vi "IslandLines.vi"(6 "Spacing":dbl, 7 "IslandSize":dbl, 8 "yMax":dbl, 9 "yMin":dbl, 10 "xMax":dbl, 11 "xMin":dbl) -> (2 "Poly2D":T1, 3 "Pnts":sgl[][](array[numeric]))   [LabVIEW 2014]
uses:
  TypeDefs/Poly2DwSlope.ctl
  TypeDefs/Point2DwSlope.ctl
panel:
  out "XY Graph":T3(graph)
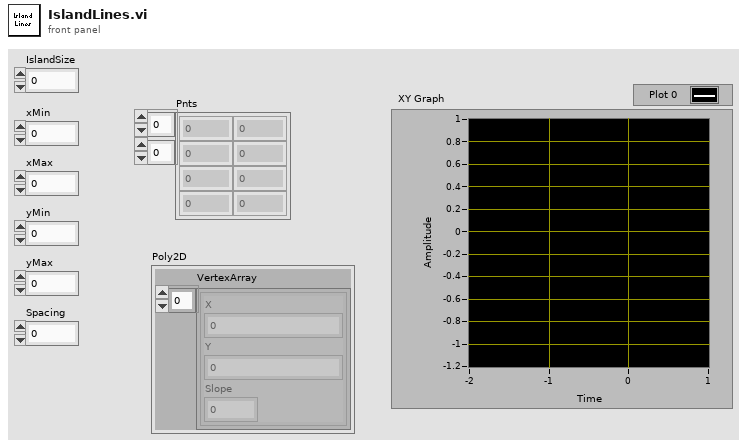
[diagram p1: front panel]
types:
  T1 = typedef "Poly2DwSlope.ctl" = cluster{"VertexArray":T2[]}
  T2 = typedef "Point2DwSlope.ctl" = cluster{"X":sgl, "Y":sgl, "Slope":dbl}
  T3 = cluster{"VertexArray":cluster{"X":sgl, "Y":sgl, "Slope":dbl}[]}[]
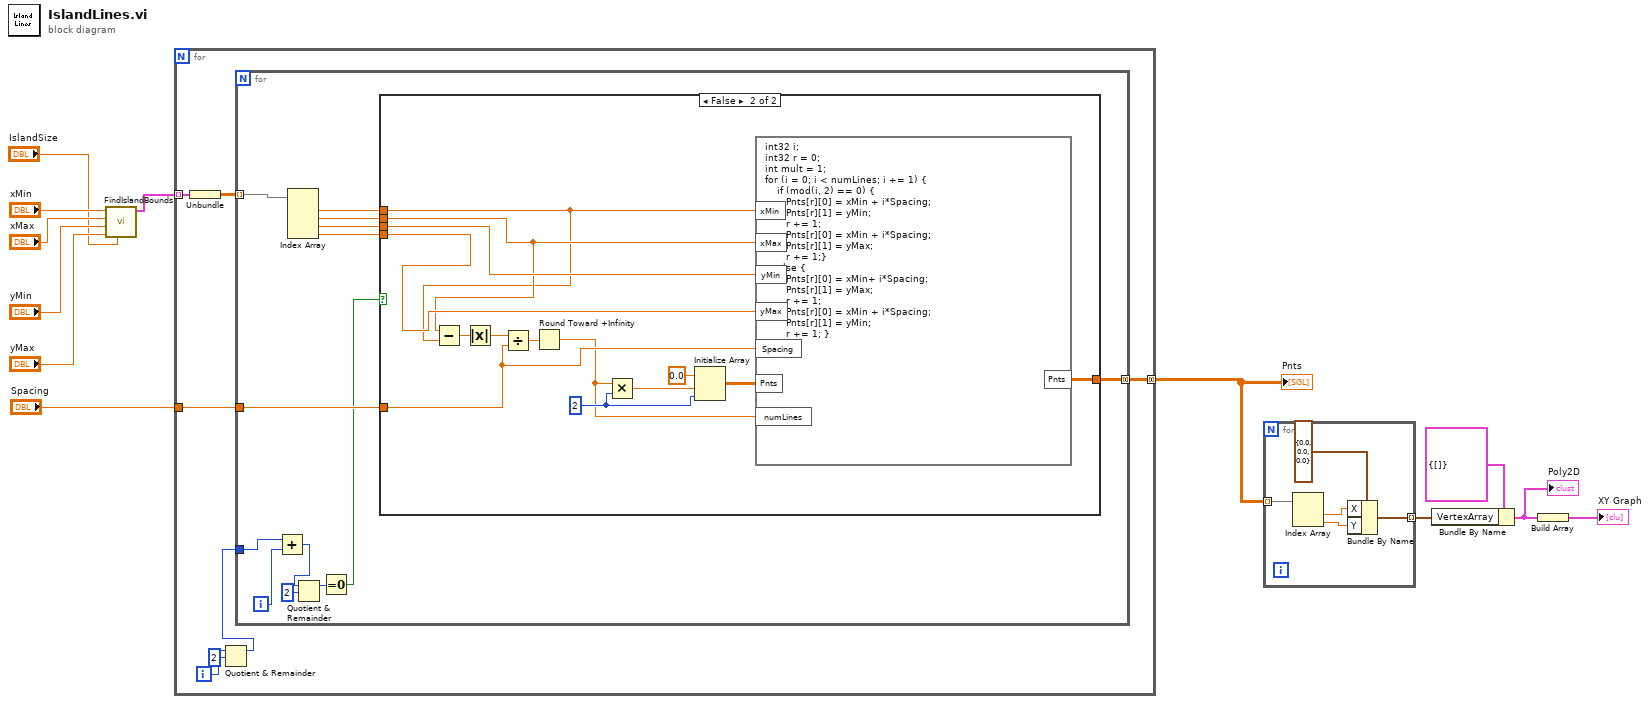
[diagram p0: block diagram]
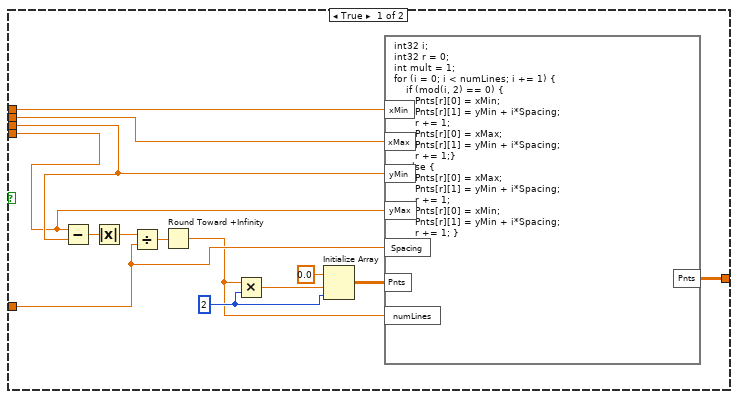
[diagram p2: hidden frame]
diagram:
  n1 = call "FindIslandBounds.vi"("IslandSize"="IslandSize", "yMax"="yMax", "yMin"="yMin", "xMax"="xMax", "xMin"="xMin") -> ("Bounds"=w2:cluster{dbl[][]}[])  [unwired: 6 in]
  n2 = for {
    tunnel: "Spacing" -> [w19]
    tunnel: [w18] -> w11 mode=concatenating
    tunnel: w2 -> [w17] mode=indexing
    i -> [w16]
    n3 = Unbundle(w17) -> (w14:dbl[][])
    n4 = Quotient & Remainder(x=w16, y=2) -> (x-y*floor(x/y)=w13:i32)  [unwired: 1 out]
    n5 = for {
      tunnel: w19 -> [w32]
      tunnel: [w31] -> w18 mode=concatenating
      tunnel: w14 -> [w30] mode=indexing
      tunnel: w13 -> [w21]
      i -> [w22]
      n6 = Add(x=w21, y=w22) -> (x+y=w20:i32)
      n7 = Index Array(array=w30) -> (element #1=w29:dbl, element #2=w28:dbl, element #3=w27:dbl, element #4=w26:dbl)  [unwired: 4 in]
      n8 = Quotient & Remainder(x=w20, y=2) -> (x-y*floor(x/y)=w25:i32)  [unwired: 1 out]
      n9 = Equal To 0?(x=w25) -> (x = 0?=w23:bool)
      n10 = case shown="False" w23 {
        tunnel: w32 -> [w39 w53]
        tunnel: [w37 w51] -> w31
        tunnel: w29 -> [w36 w47]
        tunnel: w28 -> [w35 w48]
        tunnel: w27 -> [w34 w50]
        tunnel: w26 -> [w33 w49]
        frame True {
          w41 = 2 ("dimension size")
          n11 = Subtract(x=w33, y=w34) -> (x-y=w44:dbl)
          n12 = Absolute Value(x=w44) -> (abs(x)=w43:dbl)
          n13 = Divide(x=w43, y=w39) -> (x/y=w42:dbl)
          n14 = Round Toward +Infinity(x=w42) -> (ceil(x): smallest int >= x=w38:dbl)
          n15 = Multiply(x=w38, y=w41) -> (x*y=w40:dbl)
          n16 = Initialize Array(sgl 0.0 ("element"), w40, w41) -> (w45:sgl[][])
          n17 = formula code="int32 i;\nint32 r = 0;\nint mult = 1;\nfor (i = 0; i < numLines; i += 1) {\n    if (mod(i, 2) == 0) {\n       Pnts[r][0] = xMin;\n       Pnts[r][1] = yMin + i*Spacing;\n       r += 1;\n       Pnts[r][0] = xMax;\n       Pnts[r][1] = yMin + i*Spacing;\n       r += 1;}\n    else {\n       Pnts[r][0] = xMax;\n       Pnts[r][1] = yMin + i*Spacing;\n       r += 1;\n       Pnts[r][0] = xMin;\n       Pnts[r][1] = yMin + i*Spacing;\n       r += 1; }\n    }"("xMin"=w36, "xMax"=w35, "yMin"=w34, "yMax"=w33, "Spacing"=w39, "Pnts"=w45, "numLines"=w38) -> ("Pnts"=w37:sgl[][])
        }
        frame False {
          w55 = 2 ("dimension size")
          n18 = Subtract(x=w48, y=w47) -> (x-y=w58:dbl)
          n19 = Absolute Value(x=w58) -> (abs(x)=w57:dbl)
          n20 = Divide(x=w57, y=w53) -> (x/y=w56:dbl)
          n21 = Round Toward +Infinity(x=w56) -> (ceil(x): smallest int >= x=w52:dbl)
          n22 = Multiply(x=w52, y=w55) -> (x*y=w54:dbl)
          n23 = Initialize Array(sgl 0.0 ("element"), w54, w55) -> (w59:sgl[][])
          n24 = formula code="int32 i;\nint32 r = 0;\nint mult = 1;\nfor (i = 0; i < numLines; i += 1) {\n    if (mod(i, 2) == 0) {\n       Pnts[r][0] = xMin + i*Spacing;\n       Pnts[r][1] = yMin;\n       r += 1;\n       Pnts[r][0] = xMin + i*Spacing;\n       Pnts[r][1] = yMax;\n       r += 1;}\n    else {\n       Pnts[r][0] = xMin+ i*Spacing;\n       Pnts[r][1] = yMax;\n       r += 1;\n       Pnts[r][0] = xMin + i*Spacing;\n       Pnts[r][1] = yMin;\n       r += 1; }\n    }"("xMin"=w47, "xMax"=w48, "yMin"=w50, "yMax"=w49, "Spacing"=w53, "Pnts"=w59, "numLines"=w52) -> ("Pnts"=w51:sgl[][])
        }
      }
    }
  }
  "Pnts" <- w11
  n25 = for {
    tunnel: w11 -> [w64] mode=indexing
    tunnel: [w61] -> w9 mode=indexing
    n26 = Index Array(array=w64) -> (element #1=w63:sgl, element #2=w62:sgl)  [unwired: 2 in]
    n27 = Bundle By Name(cluster=T2 {"X"=0.0, "Y"=0.0, "Slope"=0.0} ("Point2D"), "X"=w63, "Y"=w62) -> (w61:T2)
  }
  n28 = Bundle By Name(cluster=T1 {"VertexArray"=[]} ("Poly2D"), "VertexArray"=w9) -> (w7:T1)
  "Poly2D" <- w7
  n29 = Build Array(w7) -> (→"XY Graph":T1[])
